vi "Align Inline Buffer.vi"(8 "error in (no error)":errorcluster, 10 "base Inline Buffer":refnum<class "Buffer.lvclass">, 11 "Buffers in":refnum<class "Buffers.lvclass">) -> (0 "error out":errorcluster, 3 "Buffers out":refnum<class "Buffers.lvclass">)   [LabVIEW 2019, in "DSF Core.lvlib" / "Buffers.lvclass"]
uses:
  Buffers.lvclass
  Buffer/Buffer.lvclass
  C:/Program Files (x86)/National Instruments/LabVIEW 2019/vi.lib/NI/Memory Manager/Classes/Pointer/Pointer.lvclass
  Buffers.lvclass/Buffers.ctl
  <vilib>/NI/Memory Manager/Classes/Pointer/Pointer.lvclass/Pointer.ctl
  Buffer/Buffer.lvclass/Buffer.ctl
  <vilib>/NI/Memory Manager/Classes/Pointer/Get Address.vi
  <vilib>/NI/Memory Manager/Classes/Pointer/Encapsulate.vi
  <vilib>/NI/Memory Manager/Classes/Pointer/Get Size.vi
  <vilib>/NI/Memory Manager/Classes/Pointer/Is Null.vi
  <vilib>/NI/Memory Manager/Classes/Pointer/Set Size.vi
  <vilib>/NI/Memory Manager/Classes/Pointer/Set Address.vi
  <vilib>/NI/Memory Manager/Classes/Pointer/Check Null Pointer.vi
  <vilib>/NI/Memory Manager/Classes/Pointer/Set Internal.vi
  <vilib>/NI/Memory Manager/Classes/Pointer/Errors.vi
  <vilib>/NI/Memory Manager/Classes/Pointer/Null Pointer.vi
  <vilib>/NI/Memory Manager/Classes/Pointer/Create Error.vi
  <vilib>/NI/Memory Manager/VIs/New Error Cluster.vi
  <vilib>/NI/Memory Manager/VIs/New Error Cluster (512B).vi
  <vilib>/NI/Memory Manager/VIs/Set Error Status.vi
  <vilib>/NI/Memory Manager/VIs/Set Error Code.vi
  <vilib>/NI/Memory Manager/VIs/Set Error Source.vi
  <vilib>/NI/Memory Manager/Constants/Constants.vi
  <vilib>/NI/Memory Manager/Constants/Library Name.vi
  <vilib>/NI/Memory Manager/Classes/Pointer/Pointer Error Info.vi
  <vilib>/NI/Memory Manager/VIs/Write String to Source.vi
  <vilib>/NI/Memory Manager/Constants/Pointer Class Name.vi
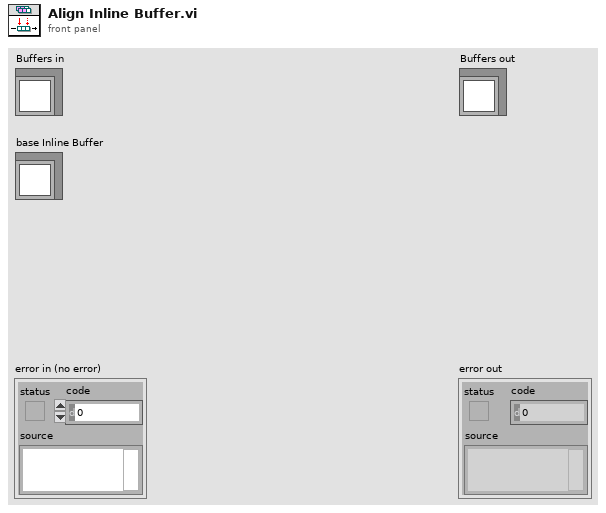
[diagram p1: front panel]
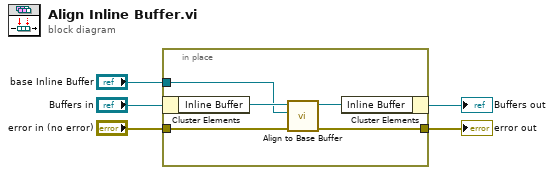
[diagram p0: block diagram]
diagram:
  n1 = in-place {
    in-place-border: [w8] -> w3
    in-place-border: "error in (no error)" -> [w7]
    in-place-border: "base Inline Buffer" -> [w6]
    n2 = in-place-cluster #1("Buffers in") -> ("Inline Buffer"=w10:refnum<class "Buffer.lvclass">)
    n3 = call "Align to Base Buffer.vi"("error in (no error)"=w7, "base Buffer"=w6, "Buffer in"=w10) -> ("error out"=w8:errorcluster, "Buffer out"=w9:refnum<class "Buffer.lvclass">)  [unwired: 7 in]
    n4 = in-place-cluster #1("Inline Buffer"=w9) -> (→"Buffers out":refnum<class "Buffers.lvclass">)
  }
  "error out" <- w3
